vi "Apply Filter.vi"(8 "error in":errorcluster, 10 "Filter Criteria":T3, 11 "Property Array":T1[](array[typedef])) -> (0 "error out":errorcluster, 3 "Filtered Property Array Out":T1[](array[typedef]))   [LabVIEW 2014]
uses:
  Controls/Property.ctl
  Controls/Address.ctl
  Controls/Filter Criteria.ctl
  Controls/Fields.ctl
  Controls/Operator.ctl
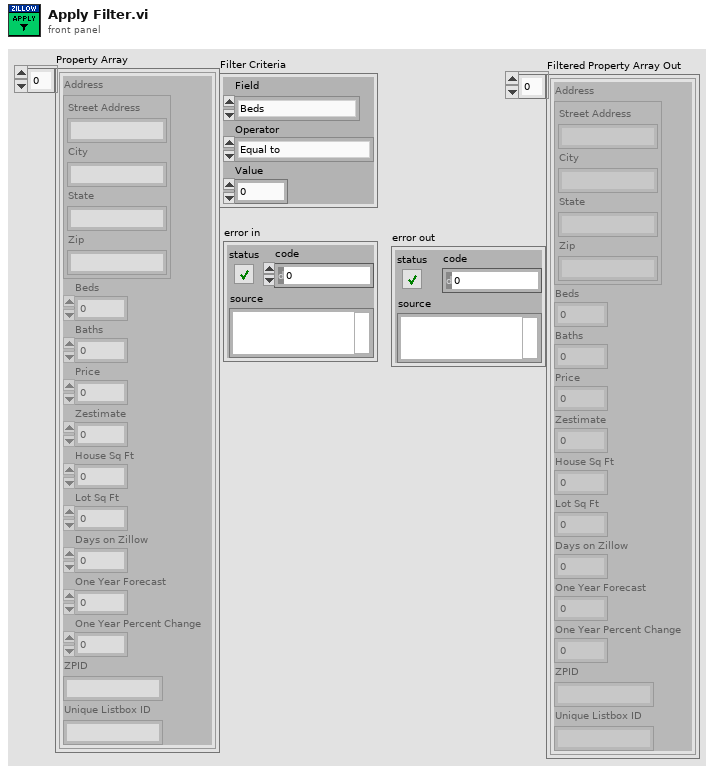
[diagram p1: front panel]
types:
  T1 = typedef "Property.ctl" = cluster{"Address":T2, "Beds":dbl, "Baths":dbl, "Price":dbl, "Zestimate":dbl, "House Sq Ft":dbl, "Lot Sq Ft":dbl, "Days on Zillow":dbl, "One Year Forecast":dbl, "One Year Percent Change":dbl, "ZPID":string, "Unique Listbox ID":string}
  T2 = typedef "Address.ctl" = cluster{"Street Address":string, "City":string, "State":string, "Zip":string}
  T3 = typedef "Filter Criteria.ctl" = cluster{"Field":T4, "Operator":T5, "Value":dbl}
  T4 = typedef "Fields.ctl" = enum16{"Beds", "Baths", "Price", "Zestimate", "House Sq Ft", "Lot Sq Ft", "Days on Zillow", "One Year Forecast", "One Year Percent Change"}
  T5 = typedef "Operator.ctl" = enum16{"Equal to", "Greater than (or equal)", "Less than (or equal)", "Not Equal to"}
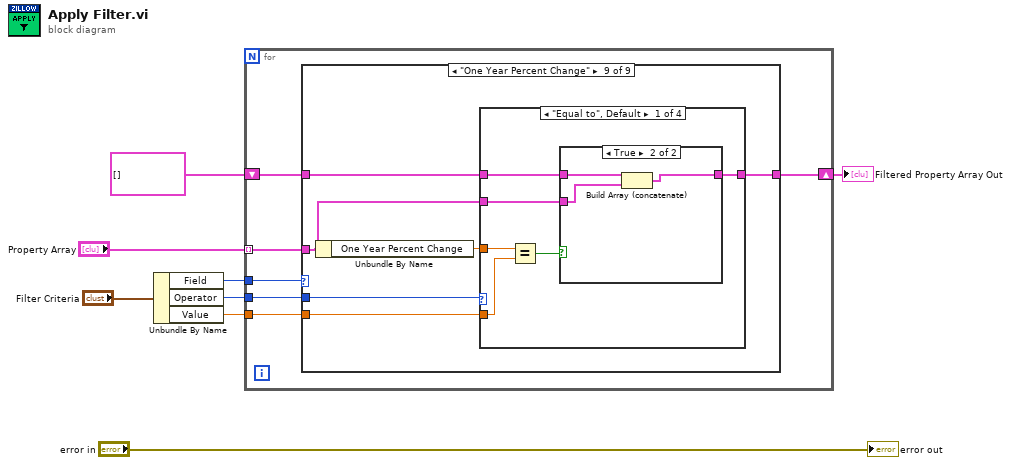
[diagram p0: block diagram]
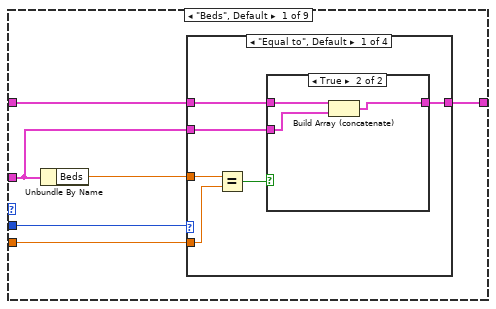
[diagram p2: hidden frame]
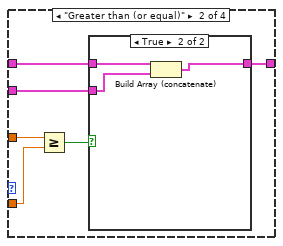
[diagram p4: hidden frame]
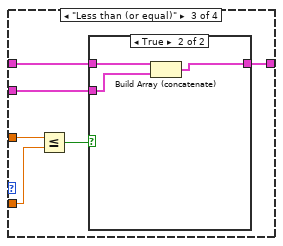
[diagram p6: hidden frame]
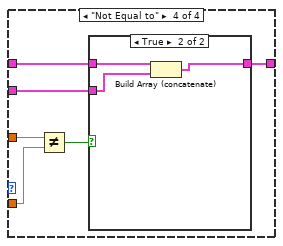
[diagram p8: hidden frame]
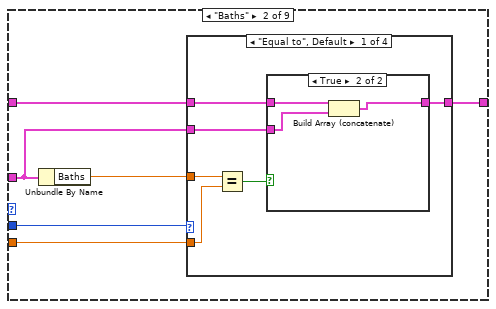
[diagram p10: hidden frame]
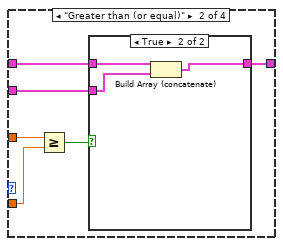
[diagram p12: hidden frame]
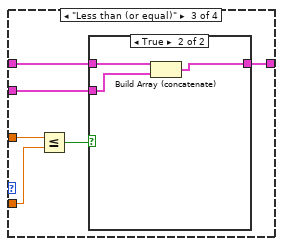
[diagram p14: hidden frame]
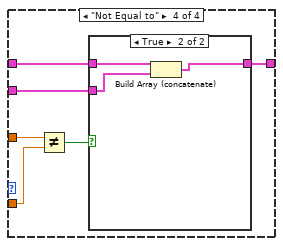
[diagram p16: hidden frame]
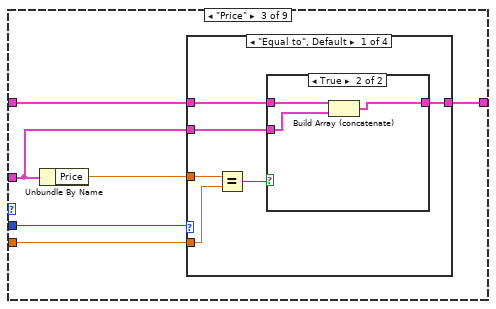
[diagram p18: hidden frame]
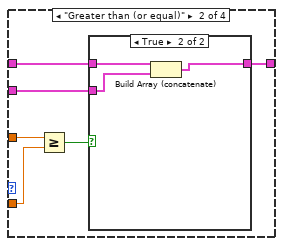
[diagram p20: hidden frame]
diagram:
  n1 = Unbundle By Name("Filter Criteria") -> ("Field"=w7:T4, "Operator"=w6:T5, "Value"=w4:dbl)
  n2 = for {
    tunnel: w7 -> [w14]
    tunnel: w6 -> [w13]
    tunnel: "Property Array" -> [w12] mode=indexing
    tunnel: w4 -> [w11]
    shift-right: [w9] -> w2
    shift-left: T1[] [] ("All Property Array") -> [w10]
    n3 = case shown="\"One Year Percent Change\"" w14 {
      tunnel: w13 -> [w20 w66 w112 w158 w204 w250 w296 w342 w388]
      tunnel: w12 -> [w16 w62 w108 w154 w200 w246 w292 w338 w384]
      tunnel: w11 -> [w18 w64 w110 w156 w202 w248 w294 w340 w386]
      tunnel: w10 -> [w17 w63 w109 w155 w201 w247 w293 w339 w385]
      tunnel: [w15 w61 w107 w153 w199 w245 w291 w337 w383] -> w9
      frame "Beds", Default {
        n4 = Unbundle By Name(w16) -> ("Beds"=w19:dbl)
        n5 = case shown="\"Equal to\", Default" w20 {
          tunnel: w19 -> [w26 w36 w46 w56]
          tunnel: w18 -> [w25 w35 w45 w55]
          tunnel: w17 -> [w23 w33 w43 w53]
          tunnel: w16 -> [w22 w32 w42 w52]
          tunnel: [w21 w31 w41 w51] -> w15
          frame "Equal to", Default {
            n6 = Equal?(x=w26, y=w25) -> (x = y?=w24:bool)
            n7 = case shown="True" w24 {
              tunnel: w23 -> [w27 w30]
              tunnel: w22 -> [_ w29]
              tunnel: [w27 w28] -> w21
              frame False {
              }
              frame True {
                n8 = Build Array (concatenate)(w30, w29) -> (w28:T1[])
              }
            }
          }
          frame "Greater than (or equal)" {
            n9 = Greater Or Equal?(x=w36, y=w35) -> (x >= y?=w34:bool)
            n10 = case shown="True" w34 {
              tunnel: w33 -> [w37 w40]
              tunnel: w32 -> [_ w39]
              tunnel: [w37 w38] -> w31
              frame False {
              }
              frame True {
                n11 = Build Array (concatenate)(w40, w39) -> (w38:T1[])
              }
            }
          }
          frame "Less than (or equal)" {
            n12 = Less Or Equal?(x=w46, y=w45) -> (x <= y?=w44:bool)
            n13 = case shown="True" w44 {
              tunnel: w43 -> [w47 w50]
              tunnel: w42 -> [_ w49]
              tunnel: [w47 w48] -> w41
              frame False {
              }
              frame True {
                n14 = Build Array (concatenate)(w50, w49) -> (w48:T1[])
              }
            }
          }
          frame "Not Equal to" {
            n15 = Not Equal?(x=w56, y=w55) -> (x != y?=w54:bool)
            n16 = case shown="True" w54 {
              tunnel: w53 -> [w57 w60]
              tunnel: w52 -> [_ w59]
              tunnel: [w57 w58] -> w51
              frame False {
              }
              frame True {
                n17 = Build Array (concatenate)(w60, w59) -> (w58:T1[])
              }
            }
          }
        }
      }
      frame "Baths" {
        n18 = Unbundle By Name(w62) -> ("Baths"=w65:dbl)
        n19 = case shown="\"Equal to\", Default" w66 {
          tunnel: w65 -> [w72 w82 w92 w102]
          tunnel: w64 -> [w71 w81 w91 w101]
          tunnel: w63 -> [w69 w79 w89 w99]
          tunnel: w62 -> [w68 w78 w88 w98]
          tunnel: [w67 w77 w87 w97] -> w61
          frame "Equal to", Default {
            n20 = Equal?(x=w72, y=w71) -> (x = y?=w70:bool)
            n21 = case shown="True" w70 {
              tunnel: w69 -> [w73 w76]
              tunnel: w68 -> [_ w75]
              tunnel: [w73 w74] -> w67
              frame False {
              }
              frame True {
                n22 = Build Array (concatenate)(w76, w75) -> (w74:T1[])
              }
            }
          }
          frame "Greater than (or equal)" {
            n23 = Greater Or Equal?(x=w82, y=w81) -> (x >= y?=w80:bool)
            n24 = case shown="True" w80 {
              tunnel: w79 -> [w83 w86]
              tunnel: w78 -> [_ w85]
              tunnel: [w83 w84] -> w77
              frame False {
              }
              frame True {
                n25 = Build Array (concatenate)(w86, w85) -> (w84:T1[])
              }
            }
          }
          frame "Less than (or equal)" {
            n26 = Less Or Equal?(x=w92, y=w91) -> (x <= y?=w90:bool)
            n27 = case shown="True" w90 {
              tunnel: w89 -> [w93 w96]
              tunnel: w88 -> [_ w95]
              tunnel: [w93 w94] -> w87
              frame False {
              }
              frame True {
                n28 = Build Array (concatenate)(w96, w95) -> (w94:T1[])
              }
            }
          }
          frame "Not Equal to" {
            n29 = Not Equal?(x=w102, y=w101) -> (x != y?=w100:bool)
            n30 = case shown="True" w100 {
              tunnel: w99 -> [w103 w106]
              tunnel: w98 -> [_ w105]
              tunnel: [w103 w104] -> w97
              frame False {
              }
              frame True {
                n31 = Build Array (concatenate)(w106, w105) -> (w104:T1[])
              }
            }
          }
        }
      }
      frame "Price" {
        n32 = Unbundle By Name(w108) -> ("Price"=w111:dbl)
        n33 = case shown="\"Equal to\", Default" w112 {
          tunnel: w111 -> [w118 w128 w138 w148]
          tunnel: w110 -> [w117 w127 w137 w147]
          tunnel: w109 -> [w115 w125 w135 w145]
          tunnel: w108 -> [w114 w124 w134 w144]
          tunnel: [w113 w123 w133 w143] -> w107
          frame "Equal to", Default {
            n34 = Equal?(x=w118, y=w117) -> (x = y?=w116:bool)
            n35 = case shown="True" w116 {
              tunnel: w115 -> [w119 w122]
              tunnel: w114 -> [_ w121]
              tunnel: [w119 w120] -> w113
              frame False {
              }
              frame True {
                n36 = Build Array (concatenate)(w122, w121) -> (w120:T1[])
              }
            }
          }
          frame "Greater than (or equal)" {
            n37 = Greater Or Equal?(x=w128, y=w127) -> (x >= y?=w126:bool)
            n38 = case shown="True" w126 {
              tunnel: w125 -> [w129 w132]
              tunnel: w124 -> [_ w131]
              tunnel: [w129 w130] -> w123
              frame False {
              }
              frame True {
                n39 = Build Array (concatenate)(w132, w131) -> (w130:T1[])
              }
            }
          }
          frame "Less than (or equal)" {
            n40 = Less Or Equal?(x=w138, y=w137) -> (x <= y?=w136:bool)
            n41 = case shown="True" w136 {
              tunnel: w135 -> [w139 w142]
              tunnel: w134 -> [_ w141]
              tunnel: [w139 w140] -> w133
              frame False {
              }
              frame True {
                n42 = Build Array (concatenate)(w142, w141) -> (w140:T1[])
              }
            }
          }
          frame "Not Equal to" {
            n43 = Not Equal?(x=w148, y=w147) -> (x != y?=w146:bool)
            n44 = case shown="True" w146 {
              tunnel: w145 -> [w149 w152]
              tunnel: w144 -> [_ w151]
              tunnel: [w149 w150] -> w143
              frame False {
              }
              frame True {
                n45 = Build Array (concatenate)(w152, w151) -> (w150:T1[])
              }
            }
          }
        }
      }
      frame "Zestimate" {
        n46 = Unbundle By Name(w154) -> ("Zestimate"=w157:dbl)
        n47 = case shown="\"Equal to\", Default" w158 {
          tunnel: w157 -> [w164 w174 w184 w194]
          tunnel: w156 -> [w163 w173 w183 w193]
          tunnel: w155 -> [w161 w171 w181 w191]
          tunnel: w154 -> [w160 w170 w180 w190]
          tunnel: [w159 w169 w179 w189] -> w153
          frame "Equal to", Default {
            n48 = Equal?(x=w164, y=w163) -> (x = y?=w162:bool)
            n49 = case shown="True" w162 {
              tunnel: w161 -> [w165 w168]
              tunnel: w160 -> [_ w167]
              tunnel: [w165 w166] -> w159
              frame False {
              }
              frame True {
                n50 = Build Array (concatenate)(w168, w167) -> (w166:T1[])
              }
            }
          }
          frame "Greater than (or equal)" {
            n51 = Greater Or Equal?(x=w174, y=w173) -> (x >= y?=w172:bool)
            n52 = case shown="True" w172 {
              tunnel: w171 -> [w175 w178]
              tunnel: w170 -> [_ w177]
              tunnel: [w175 w176] -> w169
              frame False {
              }
              frame True {
                n53 = Build Array (concatenate)(w178, w177) -> (w176:T1[])
              }
            }
          }
          frame "Less than (or equal)" {
            n54 = Less Or Equal?(x=w184, y=w183) -> (x <= y?=w182:bool)
            n55 = case shown="True" w182 {
              tunnel: w181 -> [w185 w188]
              tunnel: w180 -> [_ w187]
              tunnel: [w185 w186] -> w179
              frame False {
              }
              frame True {
                n56 = Build Array (concatenate)(w188, w187) -> (w186:T1[])
              }
            }
          }
          frame "Not Equal to" {
            n57 = Not Equal?(x=w194, y=w193) -> (x != y?=w192:bool)
            n58 = case shown="True" w192 {
              tunnel: w191 -> [w195 w198]
              tunnel: w190 -> [_ w197]
              tunnel: [w195 w196] -> w189
              frame False {
              }
              frame True {
                n59 = Build Array (concatenate)(w198, w197) -> (w196:T1[])
              }
            }
          }
        }
      }
      frame "House Sq Ft" {
        n60 = Unbundle By Name(w200) -> ("House Sq Ft"=w203:dbl)
        n61 = case shown="\"Equal to\", Default" w204 {
          tunnel: w203 -> [w210 w220 w230 w240]
          tunnel: w202 -> [w209 w219 w229 w239]
          tunnel: w201 -> [w207 w217 w227 w237]
          tunnel: w200 -> [w206 w216 w226 w236]
          tunnel: [w205 w215 w225 w235] -> w199
          frame "Equal to", Default {
            n62 = Equal?(x=w210, y=w209) -> (x = y?=w208:bool)
            n63 = case shown="True" w208 {
              tunnel: w207 -> [w211 w214]
              tunnel: w206 -> [_ w213]
              tunnel: [w211 w212] -> w205
              frame False {
              }
              frame True {
                n64 = Build Array (concatenate)(w214, w213) -> (w212:T1[])
              }
            }
          }
          frame "Greater than (or equal)" {
            n65 = Greater Or Equal?(x=w220, y=w219) -> (x >= y?=w218:bool)
            n66 = case shown="True" w218 {
              tunnel: w217 -> [w221 w224]
              tunnel: w216 -> [_ w223]
              tunnel: [w221 w222] -> w215
              frame False {
              }
              frame True {
                n67 = Build Array (concatenate)(w224, w223) -> (w222:T1[])
              }
            }
          }
          frame "Less than (or equal)" {
            n68 = Less Or Equal?(x=w230, y=w229) -> (x <= y?=w228:bool)
            n69 = case shown="True" w228 {
              tunnel: w227 -> [w231 w234]
              tunnel: w226 -> [_ w233]
              tunnel: [w231 w232] -> w225
              frame False {
              }
              frame True {
                n70 = Build Array (concatenate)(w234, w233) -> (w232:T1[])
              }
            }
          }
          frame "Not Equal to" {
            n71 = Not Equal?(x=w240, y=w239) -> (x != y?=w238:bool)
            n72 = case shown="True" w238 {
              tunnel: w237 -> [w241 w244]
              tunnel: w236 -> [_ w243]
              tunnel: [w241 w242] -> w235
              frame False {
              }
              frame True {
                n73 = Build Array (concatenate)(w244, w243) -> (w242:T1[])
              }
            }
          }
        }
      }
      frame "Lot Sq Ft" {
        n74 = Unbundle By Name(w246) -> ("Lot Sq Ft"=w249:dbl)
        n75 = case shown="\"Equal to\", Default" w250 {
          tunnel: w249 -> [w256 w266 w276 w286]
          tunnel: w248 -> [w255 w265 w275 w285]
          tunnel: w247 -> [w253 w263 w273 w283]
          tunnel: w246 -> [w252 w262 w272 w282]
          tunnel: [w251 w261 w271 w281] -> w245
          frame "Equal to", Default {
            n76 = Equal?(x=w256, y=w255) -> (x = y?=w254:bool)
            n77 = case shown="True" w254 {
              tunnel: w253 -> [w257 w260]
              tunnel: w252 -> [_ w259]
              tunnel: [w257 w258] -> w251
              frame False {
              }
              frame True {
                n78 = Build Array (concatenate)(w260, w259) -> (w258:T1[])
              }
            }
          }
          frame "Greater than (or equal)" {
            n79 = Greater Or Equal?(x=w266, y=w265) -> (x >= y?=w264:bool)
            n80 = case shown="True" w264 {
              tunnel: w263 -> [w267 w270]
              tunnel: w262 -> [_ w269]
              tunnel: [w267 w268] -> w261
              frame False {
              }
              frame True {
                n81 = Build Array (concatenate)(w270, w269) -> (w268:T1[])
              }
            }
          }
          frame "Less than (or equal)" {
            n82 = Less Or Equal?(x=w276, y=w275) -> (x <= y?=w274:bool)
            n83 = case shown="True" w274 {
              tunnel: w273 -> [w277 w280]
              tunnel: w272 -> [_ w279]
              tunnel: [w277 w278] -> w271
              frame False {
              }
              frame True {
                n84 = Build Array (concatenate)(w280, w279) -> (w278:T1[])
              }
            }
          }
          frame "Not Equal to" {
            n85 = Not Equal?(x=w286, y=w285) -> (x != y?=w284:bool)
            n86 = case shown="True" w284 {
              tunnel: w283 -> [w287 w290]
              tunnel: w282 -> [_ w289]
              tunnel: [w287 w288] -> w281
              frame False {
              }
              frame True {
                n87 = Build Array (concatenate)(w290, w289) -> (w288:T1[])
              }
            }
          }
        }
      }
      frame "Days on Zillow" {
        n88 = Unbundle By Name(w292) -> ("Days on Zillow"=w295:dbl)
        n89 = case shown="\"Equal to\", Default" w296 {
          tunnel: w295 -> [w302 w312 w322 w332]
          tunnel: w294 -> [w301 w311 w321 w331]
          tunnel: w293 -> [w299 w309 w319 w329]
          tunnel: w292 -> [w298 w308 w318 w328]
          tunnel: [w297 w307 w317 w327] -> w291
          frame "Equal to", Default {
            n90 = Equal?(x=w302, y=w301) -> (x = y?=w300:bool)
            n91 = case shown="True" w300 {
              tunnel: w299 -> [w303 w306]
              tunnel: w298 -> [_ w305]
              tunnel: [w303 w304] -> w297
              frame False {
              }
              frame True {
                n92 = Build Array (concatenate)(w306, w305) -> (w304:T1[])
              }
            }
          }
          frame "Greater than (or equal)" {
            n93 = Greater Or Equal?(x=w312, y=w311) -> (x >= y?=w310:bool)
            n94 = case shown="True" w310 {
              tunnel: w309 -> [w313 w316]
              tunnel: w308 -> [_ w315]
              tunnel: [w313 w314] -> w307
              frame False {
              }
              frame True {
                n95 = Build Array (concatenate)(w316, w315) -> (w314:T1[])
              }
            }
          }
          frame "Less than (or equal)" {
            n96 = Less Or Equal?(x=w322, y=w321) -> (x <= y?=w320:bool)
            n97 = case shown="True" w320 {
              tunnel: w319 -> [w323 w326]
              tunnel: w318 -> [_ w325]
              tunnel: [w323 w324] -> w317
              frame False {
              }
              frame True {
                n98 = Build Array (concatenate)(w326, w325) -> (w324:T1[])
              }
            }
          }
          frame "Not Equal to" {
            n99 = Not Equal?(x=w332, y=w331) -> (x != y?=w330:bool)
            n100 = case shown="True" w330 {
              tunnel: w329 -> [w333 w336]
              tunnel: w328 -> [_ w335]
              tunnel: [w333 w334] -> w327
              frame False {
              }
              frame True {
                n101 = Build Array (concatenate)(w336, w335) -> (w334:T1[])
              }
            }
          }
        }
      }
      frame "One Year Forecast" {
        n102 = Unbundle By Name(w338) -> ("One Year Forecast"=w341:dbl)
        n103 = case shown="\"Equal to\", Default" w342 {
          tunnel: w341 -> [w348 w358 w368 w378]
          tunnel: w340 -> [w347 w357 w367 w377]
          tunnel: w339 -> [w345 w355 w365 w375]
          tunnel: w338 -> [w344 w354 w364 w374]
          tunnel: [w343 w353 w363 w373] -> w337
          frame "Equal to", Default {
            n104 = Equal?(x=w348, y=w347) -> (x = y?=w346:bool)
            n105 = case shown="True" w346 {
              tunnel: w345 -> [w349 w352]
              tunnel: w344 -> [_ w351]
              tunnel: [w349 w350] -> w343
              frame False {
              }
              frame True {
                n106 = Build Array (concatenate)(w352, w351) -> (w350:T1[])
              }
            }
          }
          frame "Greater than (or equal)" {
            n107 = Greater Or Equal?(x=w358, y=w357) -> (x >= y?=w356:bool)
            n108 = case shown="True" w356 {
              tunnel: w355 -> [w359 w362]
              tunnel: w354 -> [_ w361]
              tunnel: [w359 w360] -> w353
              frame False {
              }
              frame True {
                n109 = Build Array (concatenate)(w362, w361) -> (w360:T1[])
              }
            }
          }
          frame "Less than (or equal)" {
            n110 = Less Or Equal?(x=w368, y=w367) -> (x <= y?=w366:bool)
            n111 = case shown="True" w366 {
              tunnel: w365 -> [w369 w372]
              tunnel: w364 -> [_ w371]
              tunnel: [w369 w370] -> w363
              frame False {
              }
              frame True {
                n112 = Build Array (concatenate)(w372, w371) -> (w370:T1[])
              }
            }
          }
          frame "Not Equal to" {
            n113 = Not Equal?(x=w378, y=w377) -> (x != y?=w376:bool)
            n114 = case shown="True" w376 {
              tunnel: w375 -> [w379 w382]
              tunnel: w374 -> [_ w381]
              tunnel: [w379 w380] -> w373
              frame False {
              }
              frame True {
                n115 = Build Array (concatenate)(w382, w381) -> (w380:T1[])
              }
            }
          }
        }
      }
      frame "One Year Percent Change" {
        n116 = Unbundle By Name(w384) -> ("One Year Percent Change"=w387:dbl)
        n117 = case shown="\"Equal to\", Default" w388 {
          tunnel: w387 -> [w394 w404 w414 w424]
          tunnel: w386 -> [w393 w403 w413 w423]
          tunnel: w385 -> [w391 w401 w411 w421]
          tunnel: w384 -> [w390 w400 w410 w420]
          tunnel: [w389 w399 w409 w419] -> w383
          frame "Equal to", Default {
            n118 = Equal?(x=w394, y=w393) -> (x = y?=w392:bool)
            n119 = case shown="True" w392 {
              tunnel: w391 -> [w395 w398]
              tunnel: w390 -> [_ w397]
              tunnel: [w395 w396] -> w389
              frame False {
              }
              frame True {
                n120 = Build Array (concatenate)(w398, w397) -> (w396:T1[])
              }
            }
          }
          frame "Greater than (or equal)" {
            n121 = Greater Or Equal?(x=w404, y=w403) -> (x >= y?=w402:bool)
            n122 = case shown="True" w402 {
              tunnel: w401 -> [w405 w408]
              tunnel: w400 -> [_ w407]
              tunnel: [w405 w406] -> w399
              frame False {
              }
              frame True {
                n123 = Build Array (concatenate)(w408, w407) -> (w406:T1[])
              }
            }
          }
          frame "Less than (or equal)" {
            n124 = Less Or Equal?(x=w414, y=w413) -> (x <= y?=w412:bool)
            n125 = case shown="True" w412 {
              tunnel: w411 -> [w415 w418]
              tunnel: w410 -> [_ w417]
              tunnel: [w415 w416] -> w409
              frame False {
              }
              frame True {
                n126 = Build Array (concatenate)(w418, w417) -> (w416:T1[])
              }
            }
          }
          frame "Not Equal to" {
            n127 = Not Equal?(x=w424, y=w423) -> (x != y?=w422:bool)
            n128 = case shown="True" w422 {
              tunnel: w421 -> [w425 w428]
              tunnel: w420 -> [_ w427]
              tunnel: [w425 w426] -> w419
              frame False {
              }
              frame True {
                n129 = Build Array (concatenate)(w428, w427) -> (w426:T1[])
              }
            }
          }
        }
      }
    }
  }
  "Filtered Property Array Out" <- w2
  "error out" <- "error in"
